vi "AB_820_850_Project_Source_Library.vi"(6 "dataForPrevious":T1, 7 "action":T6, 8 "error in (no error)":errorcluster, 9 "index in":i32, 10 "dataSource in":T5, 11 "buildObject":T4) -> (0 "error out":errorcluster, 1 "index out":i32, 2 "dataSource out":T5, 3 "buildObject out":T4)   [LabVIEW 2020]
doc: "Reads and writes the data to the object property bag."
uses:
  <resource>/Framework/Providers/API/ItemRef.ctl
  <vilib>/AppBuilder/RW_Project/AB_RW_Project_PropBag_Action.ctl
  <vilib>/AppBuilder/RW_Project/AB_RW_Project_Source_Data_for_Previous.ctl
  <vilib>/AppBuilder/AB_BuildType.ctl
  <vilib>/Utility/lvfile.llb/LVFileType.ctl
  <vilib>/Utility/lvfile.llb/NI_FileType.lvlib
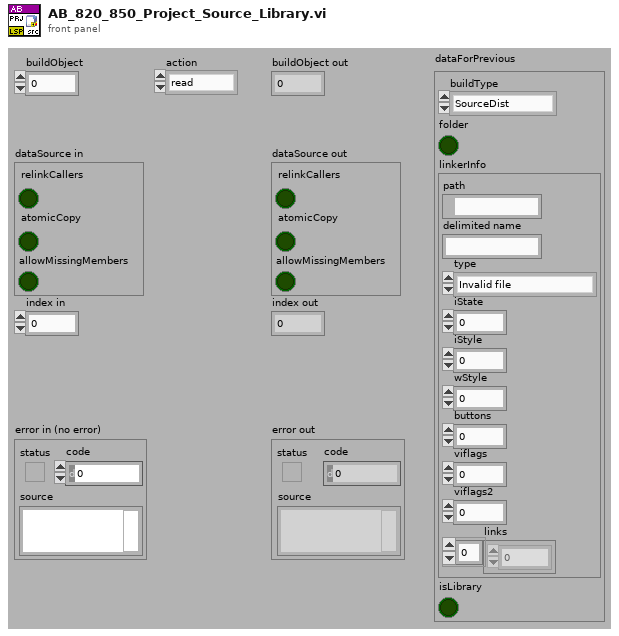
[diagram p1: front panel]
types:
  T1 = typedef "AB_RW_Project_Source_Data_for_Previous.ctl" = cluster{"buildType":T2, "folder":bool, "linkerInfo":cluster{"path":path, "delimited name":string, "type":T3, "iState":u32, "iStyle":u16, "wStyle":u16, "buttons":u16, "viflags":u32, "viflags2":u32, "links":u32[]}, "isLibrary":bool}
  T2 = typedef "AB_BuildType.ctl" = enum16{"SourceDist", "EXE", "DLL", "RTExe"}
  T3 = typedef "NI_FileType.lvlib/LVFileType.ctl" = enum32{"Invalid file", "Unknown type", "Instrument", "Control", "Polymorphic VI", "Project", "Library", "LVClass", "XControl", "XNode", "Shared library", ".NET assembly", "ActiveX interface", "CIN", "Run-time menu", "Palette menu", "Help file", "LLB", "XNode Edit Dependency", "Class Private Data Control", "Statechart", "MathScript .m file", "Ladder Diagram", "LVLibp", "XNode Build Dependency"}
  T4 = typedef "ItemRef.ctl" = u64
  T5 = cluster{"relinkCallers":bool, "atomicCopy":bool, "allowMissingMembers":bool}
  T6 = typedef "AB_RW_Project_PropBag_Action.ctl" = enum16{"read", "write", "clear", "readPrevious", "writePrevious", "clearPrevious"}
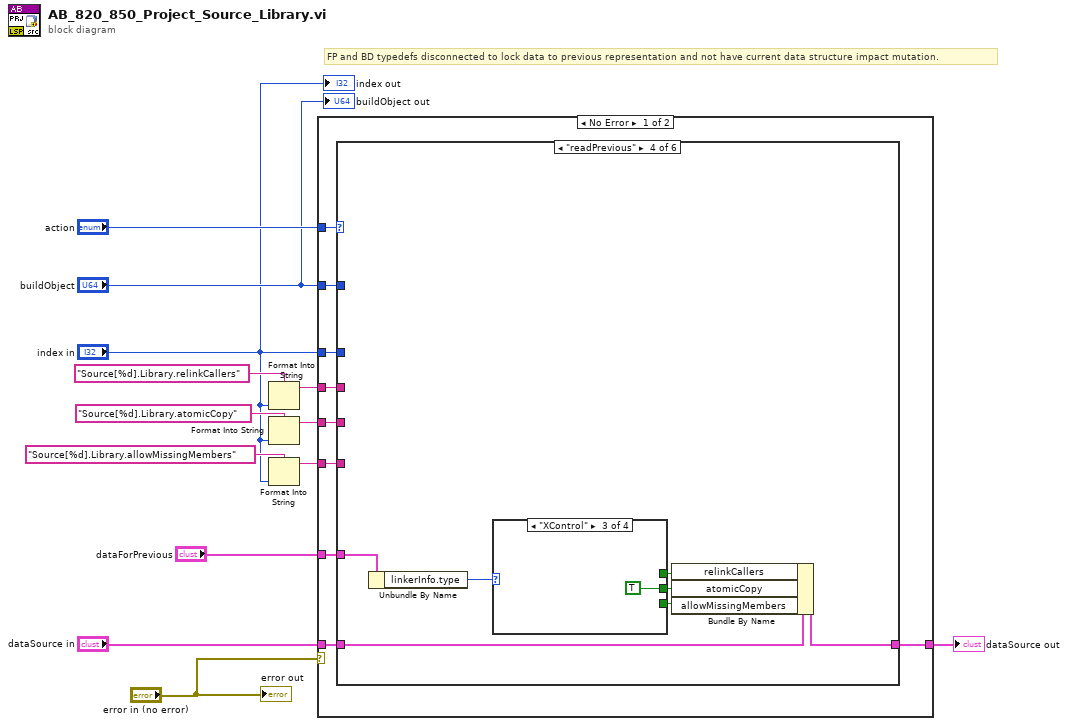
[diagram p0: block diagram]
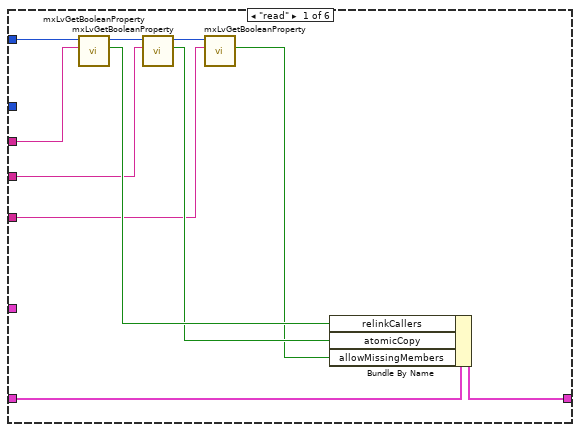
[diagram p2: hidden frame]
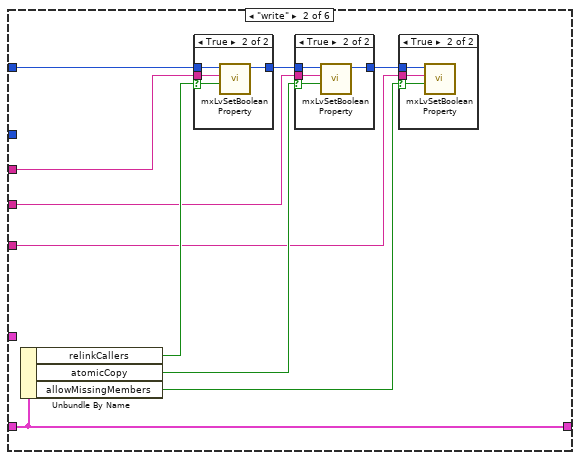
[diagram p3: hidden frame]
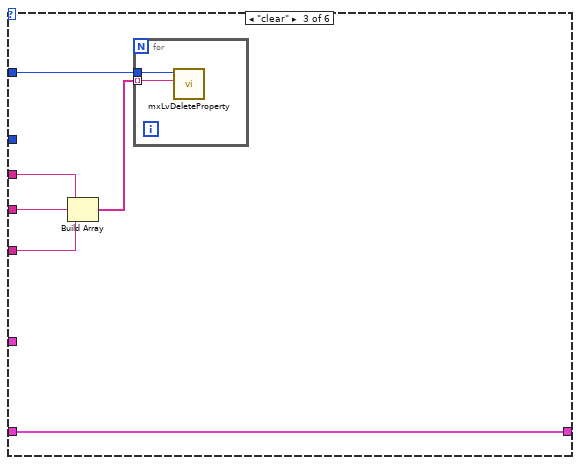
[diagram p7: hidden frame]
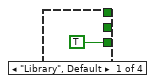
[diagram p8: hidden frame]
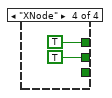
[diagram p10: hidden frame]
diagram:
  # "FP and BD typedefs disconnected to lock data to previous representation and not have current data structure impact mutation."
  n1 = Format Into String(format string="Source[%d].Library.relinkCallers", "index in") -> (resulting string=w10:string)  [unwired: 2 in, 1 out]
  n2 = Format Into String(format string="Source[%d].Library.atomicCopy", "index in") -> (resulting string=w8:string)  [unwired: 2 in, 1 out]
  n3 = Format Into String(format string="Source[%d].Library.allowMissingMembers", "index in") -> (resulting string=w1:string)  [unwired: 2 in, 1 out]
  n4 = case shown="No Error" "error in (no error)" {
    tunnel: "action" -> [w22 _]
    tunnel: "dataSource in" -> [w21 w78]
    tunnel: w10 -> [w20 _]
    tunnel: w8 -> [w19 _]
    tunnel: "index in" -> [w18 _]
    tunnel: [w17 w78] -> w7
    tunnel: "buildObject" -> [w16 _]
    tunnel: "dataForPrevious" -> [w15 _]
    tunnel: w1 -> [w14 _]
    frame No Error {
      n5 = case shown="\"readPrevious\"" w22 {
        tunnel: w16 -> [w31 w42 w58 _ _ _]
        tunnel: w21 -> [w33 w43 w62 w71 w76 w77]
        tunnel: w20 -> [w29 w40 w61 _ _ _]
        tunnel: w19 -> [w27 w38 w60 _ _ _]
        tunnel: w18 -> [_ _ _ _ _ _]
        tunnel: [w32 w43 w62 w70 w76 w77] -> w17
        tunnel: w15 -> [_ _ _ w69 _ _]
        tunnel: w14 -> [w25 w35 w57 _ _ _]
        frame "read" {
          n6 = call <resource>:"mxLvGetBooleanProperty.vi"("Tag"=w29, "Item"=w31) -> ("Value"=w30:bool, "Item"=w28:T4)  [unwired: 7 in, 1 out]
          n7 = call <resource>:"mxLvGetBooleanProperty.vi"("Tag"=w27, "Item"=w28) -> ("Value"=w26:bool, "Item"=w24:T4)  [unwired: 7 in, 1 out]
          n8 = call <resource>:"mxLvGetBooleanProperty.vi"("Tag"=w25, "Item"=w24) -> ("Value"=w23:bool)  [unwired: 7 in, 2 out]
          n9 = Bundle By Name(cluster=w33, "relinkCallers"=w30, "atomicCopy"=w26, "allowMissingMembers"=w23) -> (w32:T5)
        }
        frame "write" {
          n10 = Unbundle By Name(w43) -> ("relinkCallers"=w39:bool, "atomicCopy"=w37:bool, "allowMissingMembers"=w36:bool)
          n11 = case shown="True" w39 {
            selector: w39 -> [_ w54]
            tunnel: w42 -> [w52 w56]
            tunnel: w40 -> [_ w55]
            tunnel: [w52 w53] -> w41
            frame False {
            }
            frame True {
              n12 = call <resource>:"mxLvSetBooleanProperty.vi"("Value (F)"=w54, "Tag"=w55, "Item"=w56) -> ("Item"=w53:T4)  [unwired: 7 in, 1 out]
            }
          }
          n13 = case shown="True" w37 {
            selector: w37 -> [_ w49]
            tunnel: w41 -> [w47 w51]
            tunnel: w38 -> [_ w50]
            tunnel: [w47 w48] -> w34
            frame False {
            }
            frame True {
              n14 = call <resource>:"mxLvSetBooleanProperty.vi"("Value (F)"=w49, "Tag"=w50, "Item"=w51) -> ("Item"=w48:T4)  [unwired: 7 in, 1 out]
            }
          }
          n15 = case shown="True" w36 {
            selector: w36 -> [_ w44]
            tunnel: w34 -> [_ w46]
            tunnel: w35 -> [_ w45]
            frame False {
            }
            frame True {
              n16 = call <resource>:"mxLvSetBooleanProperty.vi"("Value (F)"=w44, "Tag"=w45, "Item"=w46) -> ()  [unwired: 7 in, 2 out]
            }
          }
        }
        frame "clear" {
          n17 = Build Array(w61, w60, w57) -> (w59:string[])
          n18 = for {
            tunnel: w58 -> [w64]
            tunnel: w59 -> [w63] mode=indexing
            n19 = call <resource>:"mxLvDeleteProperty.vi"("Tag"=w63, "Item"=w64) -> ()  [unwired: 8 in, 2 out]
          }
        }
        frame "readPrevious" {
          n20 = Unbundle By Name(w69) -> ("linkerInfo.type"=w68:T3)
          n21 = case shown="\"XControl\"" w68 {
            tunnel: [_ _ _ TRUE] -> w67
            tunnel: [_ _ TRUE TRUE] -> w66
            tunnel: [TRUE _ _ _] -> w65
            frame "Library", Default {
            }
            frame "LVClass" {
            }
            frame "XControl" {
            }
            frame "XNode" {
            }
          }
          n22 = Bundle By Name(cluster=w71, "relinkCallers"=w67, "atomicCopy"=w66, "allowMissingMembers"=w65) -> (w70:T5)
        }
        frame "writePrevious" {
        }
        frame "clearPrevious" {
        }
      }
    }
    frame Error {
    }
  }
  "dataSource out" <- w7
  "error out" <- "error in (no error)"
  "buildObject out" <- "buildObject"
  "index out" <- "index in"
